vi "Obs_init.vi"(8 "error in":errorcluster, 9 "BG_ref":refnum<vi>[](array[refnum]), 10 "ObsD_in":refnum<vi>[](array[refnum]), 11 "ObsU_in":refnum<vi>[](array[refnum])) -> (0 "error IO":errorcluster)   [LabVIEW 8.6]
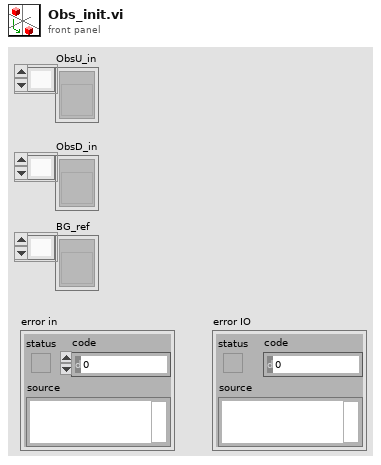
[diagram p1: front panel]
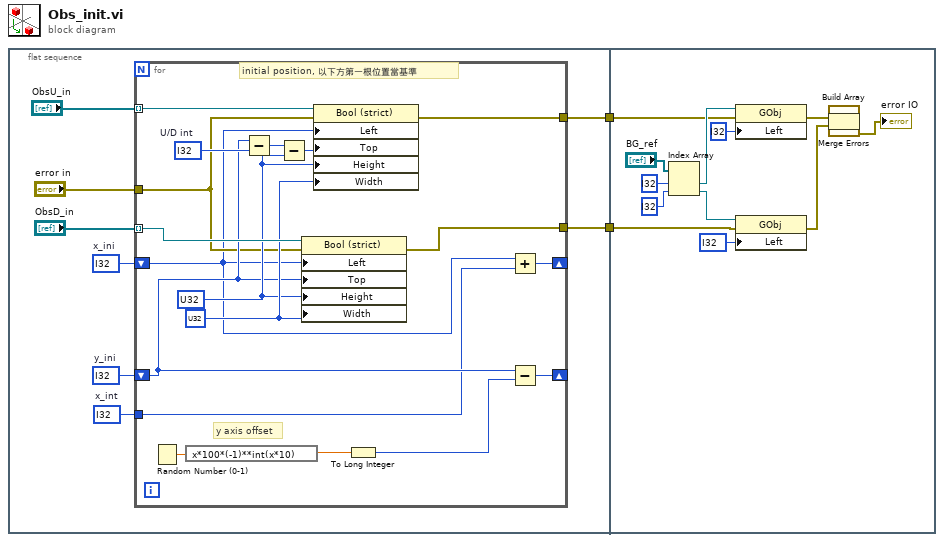
[diagram p0: block diagram]
diagram:
  n1 = flat-sequence {
    tunnel: [w4] -> w2
    tunnel: [w3] -> w1
    tunnel: w2 -> [w34]
    tunnel: w1 -> [w33]
    frame #0 {
      w5 = i32 ?  # x_int
      w10 = i32 ?  # y_ini
      w8 = i32 ?  # x_ini
      n2 = for {
        tunnel: "ObsD_in" -> [w28] mode=indexing
        shift-right: [w27] -> _
        shift-left: w8 -> [w17]
        tunnel: "ObsU_in" -> [w26] mode=indexing
        shift-right: [w20] -> _
        shift-left: w10 -> [w19]
        tunnel: "error in" -> [w18]
        tunnel: [w11] -> w4
        tunnel: w5 -> [w16]
        tunnel: [w12] -> w3
        w21 = i32 ?  # U/D int
        w25 = u32 ? ("Button Size:Width")
        w23 = u32 ? ("Button Size:Height")
        # "y axis offset"
        # "initial position, 以下方第一根位置當基準"
        n3 = Random Number (0-1)() -> (number: 0 to 1=w14:dbl)
        n4 = expression code="x*100*(-1)**int(x*10)"(w14) -> (w15:dbl)
        n5 = Subtract(x=w19, y=w21) -> (x-y=w22:i32)
        n6 = Subtract(x=w22, y=w23) -> (x-y=w24:u32)
        n7 = property on="Property Node" class="Bool (strict)"(reference=w28, error in=w18, "Left"=w17, "Top"=w19, "Height"=w23, "Width"=w25) -> (error out=w12:errorcluster)  [unwired: 1 out]
        n8 = property on="Property Node" class="Bool (strict)"(reference=w26, error in=w18, "Left"=w17, "Top"=w24, "Height"=w23, "Width"=w25) -> (error out=w11:errorcluster)  [unwired: 1 out]
        n9 = To Long Integer(number=w15) -> (32bit integer=w13:i32)
        n10 = Add(x=w17, y=w16) -> (x+y=w27:i32)
        n11 = Subtract(x=w19, y=w13) -> (x-y=w20:i32)
      }
    }
    frame #1 {
      n12 = Index Array(array="BG_ref", index #1=i32 ? ("index"), index #2=i32 ? ("index")) -> (element #1=w38:refnum<vi>, element #2=w40:refnum<vi>)
      n13 = property on="Property Node" class="GObj"(reference=w38, error in=w34, "Left"=i32 ? ("Position:Left")) -> (error out=w32:errorcluster)  [unwired: 1 out]
      n14 = property on="Property Node" class="GObj"(reference=w40, error in=w33, "Left"=i32 ? ("Position:Left")) -> (error out=w31:errorcluster)  [unwired: 1 out]
      n15 = Build Array(w32, w31) -> (w29:errorcluster[])
      n16 = call <vilib>:"Merge Errors.vi"("error array in"=w29) -> ("error out"=→"error IO":errorcluster)  [unwired: 6 in]
    }
  }
